vi "Read database.vi"(0 "condition":string="([数据标识] = 'N' or  [数据标识] = 'L') ", 1 "显示项":string[](array[string])=["top 100 *"], 5 "Table":string(combo)="CODMn", 7 "量程下拉列表":enum16{"低量程", "高量程"}(ring), 9 "量程筛选":bool, 11 "error in (no error)":errorcluster caption="错误输入（无错误）") -> (4 "表格":string[][](table), 6 "columns":string[](array[string]), 8 "foretime":string, 10 "lasttime":string, 15 "error out":errorcluster caption="错误输出")   [LabVIEW 2016]
uses:
  <vilib>/addons/database/Connection.llb/DB Tools Open Connec (String).vi
  <userlib>/_LVST/sqlite_api/Core/Tables/SQLite_List Columns.vi
  <vilib>/addons/database/_DB Variant To Data/Database Variant To Data.xnode
  <vilib>/addons/database/NI_Database_API.lvlib
  database/Access/Access Lib.lvlib
  database/SQLite/SQLite Lib.lvlib
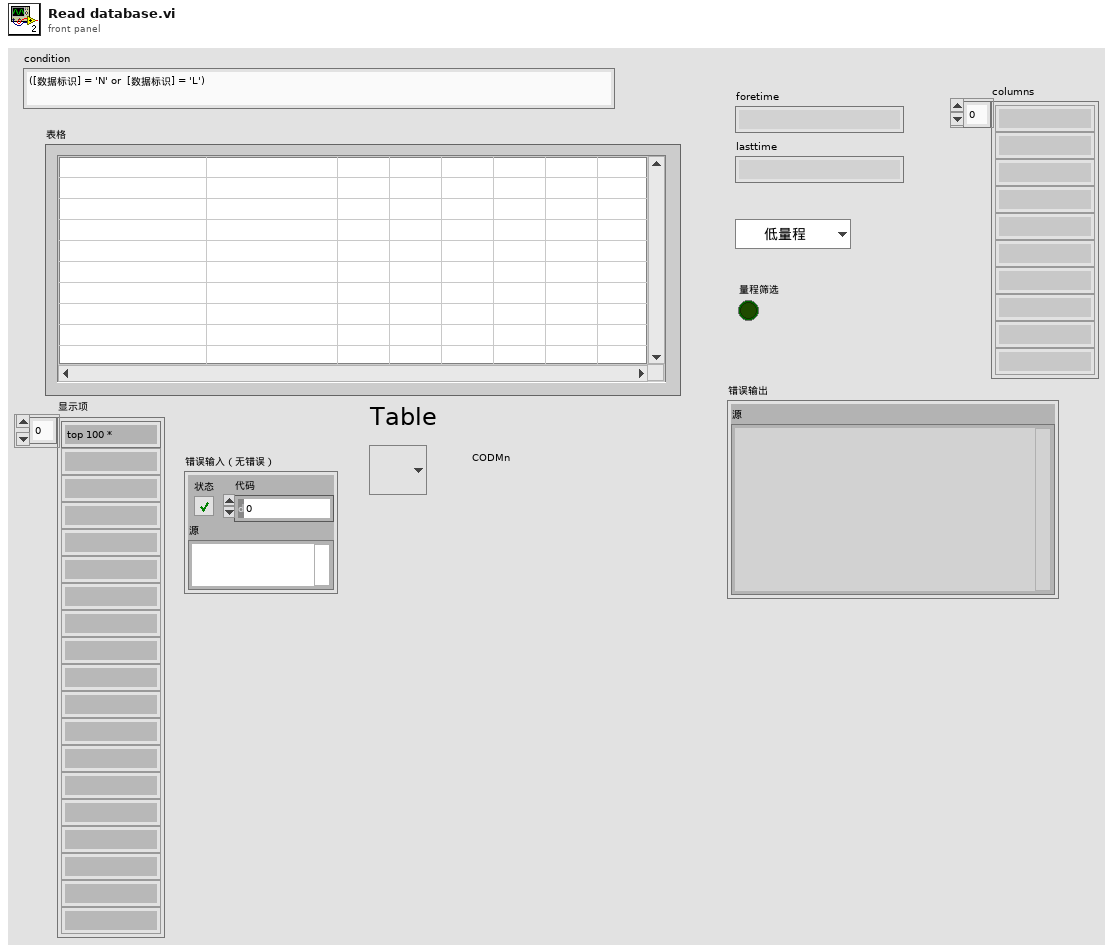
[diagram p1: front panel]
types:
  T1 = typedef "数据库类型.ctl" = enum16{"Access", "SQLite"}
  T2 = typedef "NI_Database_API.lvlib/Conn ObjectReference.ctl" = refnum<k1>
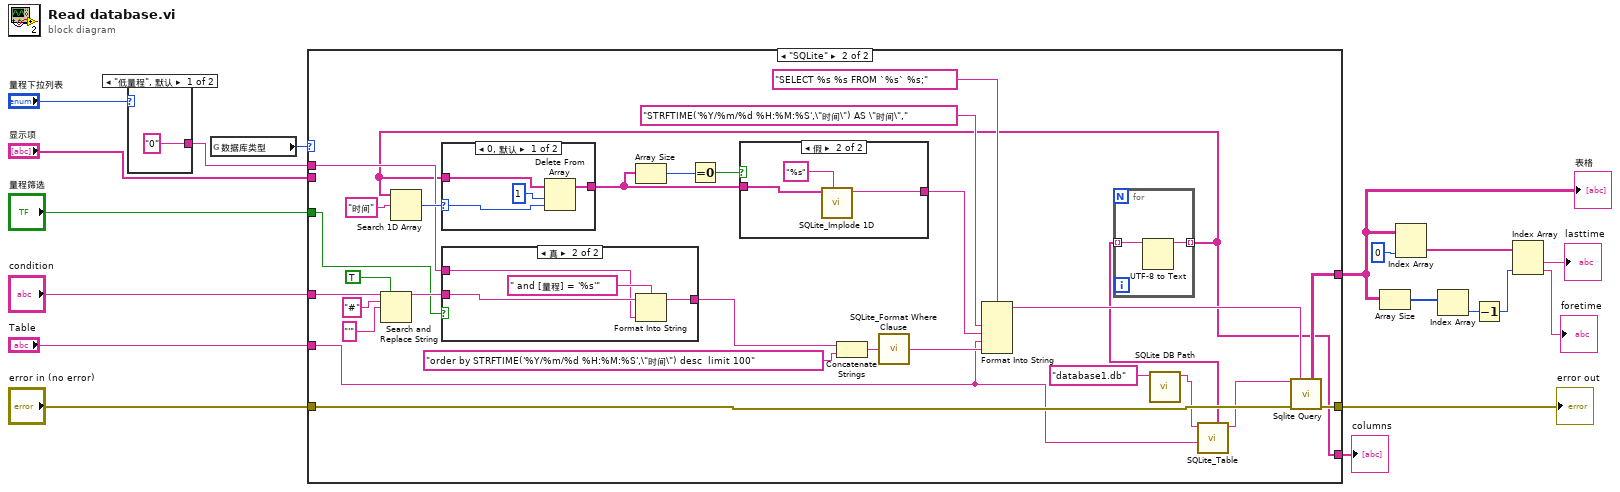
[diagram p0: block diagram]
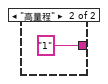
[diagram p2: hidden frame]
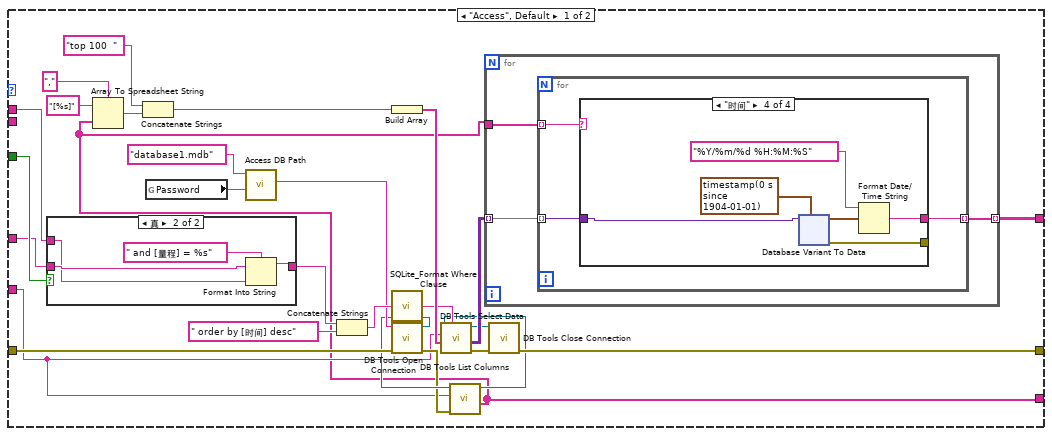
[diagram p3: hidden frame]
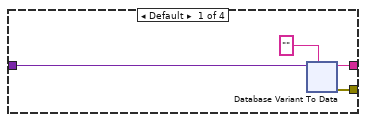
[diagram p5: hidden frame]
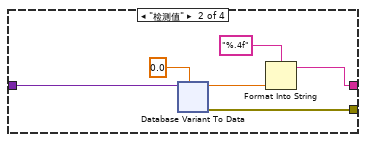
[diagram p6: hidden frame]
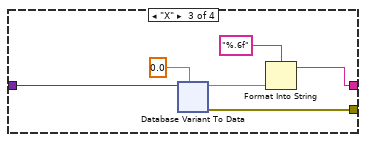
[diagram p7: hidden frame]
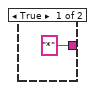
[diagram p10: hidden frame]
diagram:
  n1 = case shown="\"低量程\", 默认" "量程下拉列表" {
    tunnel: ["0" "1"] -> w3
    frame "低量程", Default {
    }
    frame "高量程" {
    }
  }
  n2 = global read "CODMn断电保存全局变量.vi" "数据库类型"() -> (w18:T1)
  n3 = case shown="\"SQLite\"" w18 {
    tunnel: "condition" -> [w28 w249]
    tunnel: "显示项" -> [_ _]
    tunnel: "Table" -> [w23 w224]
    tunnel: "error in (no error)" -> [w42 w236]
    tunnel: [w34 w235] -> w15
    tunnel: [w33 w231] -> w9
    tunnel: w3 -> [w30 w229]
    tunnel: "量程筛选" -> [w29 w227]
    tunnel: [w21 w222] -> w1
    frame "Access", Default {
      n4 = case shown="真" w29 {
        tunnel: w28 -> [w48 w52]
        tunnel: [w48 w51] -> w31
        tunnel: w30 -> [_ w50]
        frame False {
        }
        frame True {
          n5 = Format Into String(format string=" and [量程] = %s" ("格式字符串"), initial string=w52, w50) -> (resulting string=w51:string)  [unwired: 1 in, 1 out]
        }
      }
      n6 = global read "CODMn断电保存全局变量.vi" "Password"() -> (w26:string)
      n7 = call "Access DB Path.vi"("Password"=w26, "database"="database1.mdb") -> ("Connection information"=w27:string)  [unwired: 8 in, 1 out]
      n8 = Concatenate Strings(w31, " order by [时间] desc" ("字符串")) -> (w46:string)
      n9 = call <userlib>:"SQLite_Format Where Clause.vi"("Where clause"=w46) -> ("String"=w32:string)  [unwired: 4 in]
      n10 = call-poly <vilib>:"DB Tools Open Connection.vi"("error in (no error)"=w42, "connection information"=w27) -> ("error out"=w24:errorcluster, "connection reference"=w25:T2)  [unwired: 6 in]
      n11 = call <vilib>:"DB Tools List Columns.vi"("error in (no error)"=w24, "table"=w23, "connection reference"=w25) -> ("columns"=w21:string[], "connection reference out"=w22:T2)  [unwired: 1 in, 2 out]
      n12 = Array To Spreadsheet String(delimiter (Tab)="," ("分隔符(Tab)"), array=w21, 3:"[%s]" ("格式字符串")) -> (spreadsheet string=w40:string)
      n13 = Concatenate Strings("top 100  " ("字符串"), w40) -> (w39:string)
      n14 = Build Array(w39) -> (w38:string[])
      n15 = call <vilib>:"DB Tools Select Data.vi"("condition"=w32, "columns"=w38, "table"=w23, "connection reference"=w22) -> ("error out"=w35:errorcluster, "data"=w37:variant[][], "connection reference out"=w36:T2)  [unwired: 2 in]
      n16 = for {
        tunnel: w37 -> [w55] mode=indexing
        tunnel: [w54] -> w33 mode=indexing
        tunnel: w21 -> [w53]
        n17 = for {
          tunnel: w55 -> [w57] mode=indexing
          tunnel: [w58] -> w54 mode=indexing
          tunnel: w53 -> [w56] mode=indexing
          n18 = case shown="\"时间\"" w56 {
            tunnel: w57 -> [w62 w100 w138 w176]
            tunnel: [w59 w96 w134 w172] -> w58
            tunnel: [w60 w99 w137 w171] -> _
            frame Default {
              n19 = xnode "Database Variant To Data"("database variant"=w62, "type"="") -> ("data"=w59:string, "error out"=w60:errorcluster)  [unwired: 1 in]
            }
            frame "检测值" {
              n20 = xnode "Database Variant To Data"("database variant"=w100, "type"=0.0) -> ("data"=w97:dbl, "error out"=w99:errorcluster)  [unwired: 1 in]
              n21 = Format Into String(format string="%.4f" ("格式字符串"), w97) -> (resulting string=w96:string)  [unwired: 2 in, 1 out]
            }
            frame "X" {
              n22 = xnode "Database Variant To Data"("database variant"=w138, "type"=0.0) -> ("data"=w135:dbl, "error out"=w137:errorcluster)  [unwired: 1 in]
              n23 = Format Into String(format string="%.6f" ("格式字符串"), w135) -> (resulting string=w134:string)  [unwired: 2 in, 1 out]
            }
            frame "时间" {
              n24 = xnode "Database Variant To Data"("database variant"=w176, "type"=timestamp(0 s since 1904-01-01) ("当前时间")) -> ("data"=w175:timestamp, "error out"=w171:errorcluster)  [unwired: 1 in]
              n25 = Format Date/Time String(time format string (%c)="%Y/%m/%d %H:%M:%S" ("时间格式字符串(%c)"), seconds (now)=w175) -> (date/time string=w172:string)  [unwired: 1 in]
            }
          }
        }
      }
      n26 = call <vilib>:"DB Tools Close Connection.vi"("error in (no error)"=w35, "connection reference"=w36) -> ("error out"=w34:errorcluster)  [unwired: 5 in]
    }
    frame "SQLite" {
      n27 = Search and Replace String(replace all?=TRUE ("替换全部？(F)"), input string=w249, search string="#" ("搜索字符串"), replace string="'" ("替换字符串(\"\")")) -> (result string=w238:string)  [unwired: 4 in, 3 out]
      n28 = case shown="真" w227 {
        tunnel: w238 -> [w253 w257]
        tunnel: [w253 w256] -> w230
        tunnel: w229 -> [_ w254]
        frame False {
        }
        frame True {
          n29 = Format Into String(format string=" and [量程] = '%s'" ("格式字符串"), initial string=w257, w254) -> (resulting string=w256:string)  [unwired: 1 in, 1 out]
        }
      }
      n30 = Concatenate Strings(w230, "order by STRFTIME('%Y/%m/%d %H:%M:%S',\"时间\") desc  limit 100") -> (w234:string)
      n31 = call <userlib>:"SQLite_Format Where Clause.vi"("Where clause"=w234) -> ("String"=w233:string)  [unwired: 4 in]
      n32 = call "SQLite DB Path.vi"("database"="database1.db") -> ("Path out"=w226:string)  [unwired: 10 in]
      n33 = call-poly <userlib>:"SQLite_Table.vi"("DB Path"=w226, "Table Name"=w224) -> ("Columns"=w223:string[], "DB Path Out"=w225:string)  [unwired: 5 in, 2 out]
      n34 = for {
        tunnel: w223 -> [w252] mode=indexing
        tunnel: [w251] -> w222 mode=indexing
        n35 = UTF-8 to Text(11:w252) -> (3:w251:string)  [unwired: 2 in, 1 out]
      }
      n36 = Search 1D Array(1D array=w222, element="时间" ("元素")) -> (index of element=w242:i32)  [unwired: 1 in]
      n37 = case shown="0, 默认" w242 {
        selector: w242 -> [w260 _]
        tunnel: w222 -> [w261 w262]
        tunnel: [w258 w262] -> w243
        frame 0, Default {
          n38 = Delete From Array(array=w261, length=1 ("长度"), index=w260) -> (array with subset deleted=w258:string[])  [unwired: 1 out]
        }
        frame -1 {
        }
      }
      n39 = Array Size(array=w243) -> (size(s)=w239:i32)
      n40 = Equal To 0?(x=w239) -> (x = 0?=w240:bool)
      n41 = case shown="假" w240 {
        tunnel: w243 -> [_ w265]
        tunnel: ["*" ("t") w264] -> w232
        frame True {
        }
        frame False {
          n42 = call <userlib>:"SQLite_Implode 1D.vi"("Values"=w265, "format string"="%s") -> ("imploded string"=w264:string)  [unwired: 7 in, 1 out]
        }
      }
      n43 = Format Into String(format string="SELECT %s %s FROM `%s` %s;" ("SQL Query"), "STRFTIME('%Y/%m/%d %H:%M:%S',\"时间\") AS \"时间\",", w232, w224, w233) -> (resulting string=w228:string)  [unwired: 2 in, 1 out]
      n44 = call "Sqlite Query.vi"("DB Path"=w225, "SQL Query"=w228, "error in (no error)"=w236) -> ("Results"=w231:string[][], "error out"=w235:errorcluster)  [unwired: 10 in, 1 out]
    }
  }
  "表格" <- w9
  "error out" <- w15
  "columns" <- w1
  n45 = Array Size(array=w9) -> (size(s)=w12:i32[])
  n46 = Index Array(array=w9, index (col)=0 ("禁用的索引 (列)")) -> (element=w13:string[])  [unwired: 1 in]
  n47 = Index Array(array=w12) -> (element=w11:i32)  [unwired: 1 in]
  n48 = Decrement(x=w11) -> (x-1=w10:i32)
  n49 = Index Array(array=w13, index #2=w10) -> (element #1=→"lasttime":string, element #2=→"foretime":string)  [unwired: 1 in]
